vi "Update Boolean Value.vi"(9 "Value":bool, 10 "Tree Tag":string, 11 "Settings In":T1) -> (3 "Settings Out":T1)   [LabVIEW 2024, in "Sequencer with Output Values.lvlib" / "Sequencer with Output Values.lvclass"]
uses:
  Sequencer with Output Values.lvclass
  Params.ctl
  Step Settings.ctl
  Global Tree Data.vi
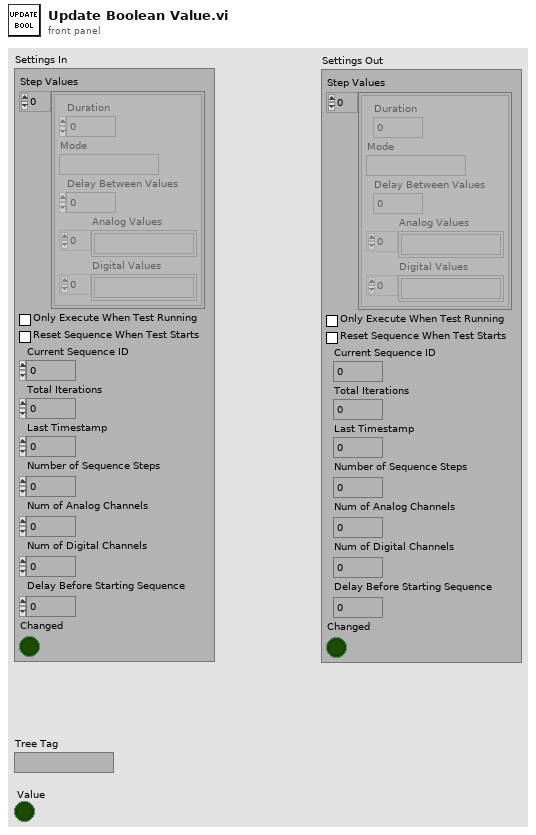
[diagram p1: front panel]
types:
  T1 = typedef "Sequencer with Output Values.lvlib/Sequencer with Output Values.lvclass/Params.ctl" = cluster{"Step Values":T2[], "Only Execute When Test Running":bool, "Reset Sequence When Test Starts":bool, "Current Sequence ID":u32, "Total Iterations":u32, "Last Timestamp":dbl, "Number of Sequence Steps":i32, "Num of Analog Channels":i32, "Num of Digital Channels":i32, "Delay Before Starting Sequence":dbl, "Changed":bool}
  T2 = typedef "Sequencer with Output Values.lvlib/Sequencer with Output Values.lvclass/Step Settings.ctl" = cluster{"Duration":dbl, "Mode":string, "Delay Between Values":dbl, "Analog Values":string[], "Digital Values":string[]}
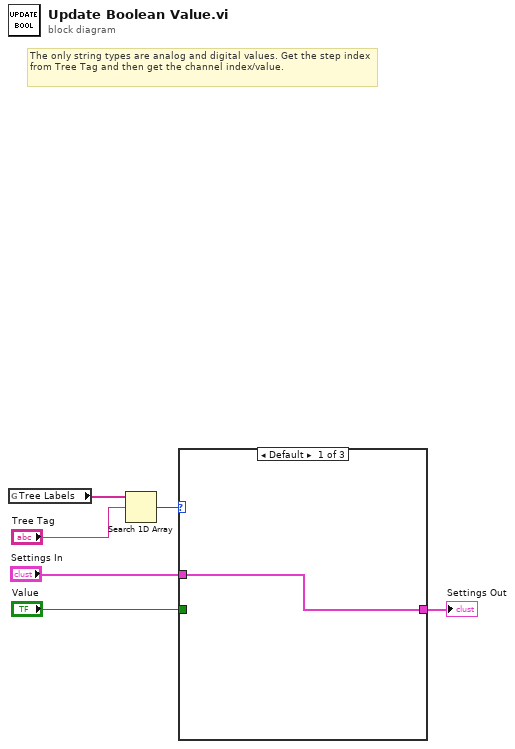
[diagram p0: block diagram]
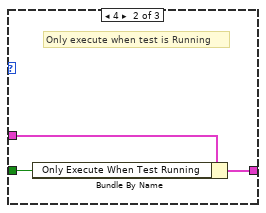
[diagram p2: hidden frame]
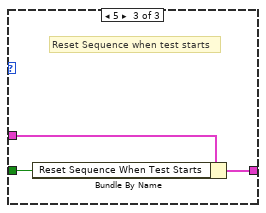
[diagram p3: hidden frame]
diagram:
  # "The only string types are analog and digital values. Get the step index from Tree Tag and then get the channel index/value."
  n1 = global read "Global Tree Data.vi" "Tree Labels"() -> (w6:string[])
  n2 = Search 1D Array(1D array=w6, element="Tree Tag") -> (index of element=w4:i32)  [unwired: 1 in]
  n3 = case shown="Default" w4 {
    tunnel: "Settings In" -> [w7 w10 w13]
    tunnel: "Value" -> [_ w9 w12]
    tunnel: [w7 w8 w11] -> w1
    frame Default {
    }
    frame 4 {
      # "Only execute when test is Running"
      n4 = Bundle By Name(cluster=w10, "Only Execute When Test Running"=w9) -> (w8:T1)
    }
    frame 5 {
      # "Reset Sequence when test starts"
      n5 = Bundle By Name(cluster=w13, "Reset Sequence When Test Starts"=w12) -> (w11:T1)
    }
  }
  "Settings Out" <- w1
